vi "Write Glue Speed.vi"(8 "error in (no error)":errorcluster, 10 "Glue Speed":i32=15, 11 "CAD Dispense in":refnum<class "Sensor Dispense.lvclass">) -> (0 "error out":errorcluster, 3 "CAD Dispense out":refnum<class "Sensor Dispense.lvclass">)   [LabVIEW 2016, in "Sensor Dispense.lvclass"]
uses:
  Sensor Dispense.lvclass
  Sensor Dispense.lvclass/Sensor Dispense.ctl
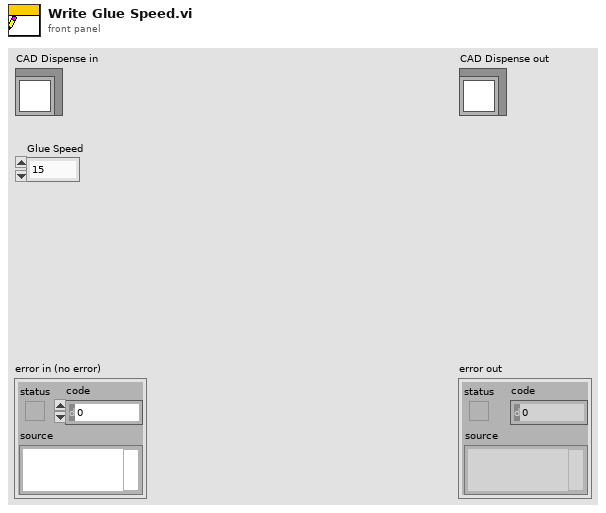
[diagram p1: front panel]
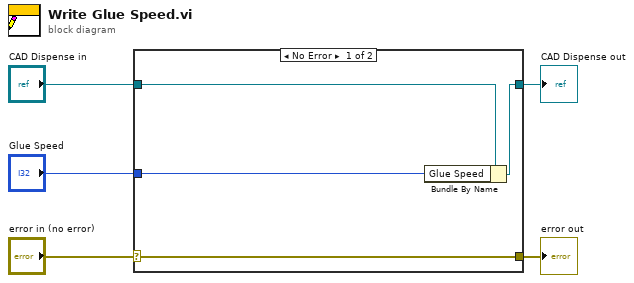
[diagram p0: block diagram]
diagram:
  n1 = case shown="No Error" "error in (no error)" {
    selector: "error in (no error)" -> [w9 w10]
    tunnel: [w9 w10] -> w4
    tunnel: [w7 w11] -> w2
    tunnel: "CAD Dispense in" -> [w8 w11]
    tunnel: "Glue Speed" -> [w6 _]
    frame No Error {
      n2 = Bundle By Name(cluster=w8, "Glue Speed"=w6) -> (w7:refnum<class "Sensor Dispense.lvclass">)
    }
    frame Error {
    }
  }
  "error out" <- w4
  "CAD Dispense out" <- w2
